vi "CC Observation List to Table.vi"(8 "error in (no error)":errorcluster, 11 "Observation List":T2[](array[typedef])) -> (0 "error out":errorcluster, 1 "Screen Ready Table":string[][](array[string]), 2 "Status":T1[](array[typedef]), 3 "File Ready Table":string[][](array[string]))   [LabVIEW 2024]
uses:
  typedefs/CC cluster Observation.ctl
  Observation Queue/CC enum Observation Status.ctl
  Telescope/CC cluster Telescope Offsets.ctl
  typedefs/CC cluster Observation Dither Options.ctl
  typedefs/CC enum Dither Selection.ctl
  typedefs/CC cluster RA and DEC.ctl
panel:
  out "Header":string[](array[string])
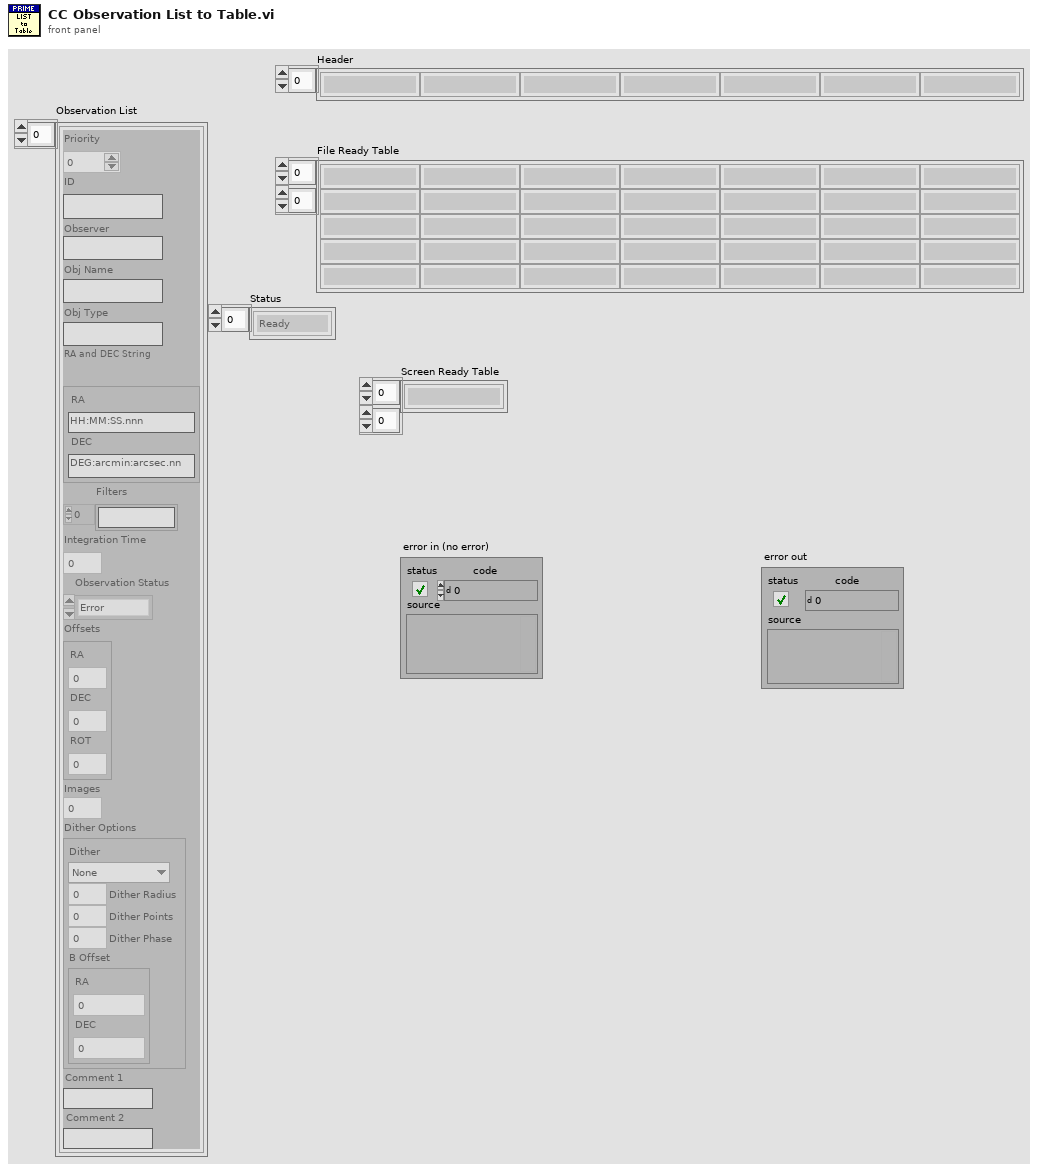
[diagram p1: front panel]
types:
  T1 = typedef "CC enum Observation Status.ctl" = enum16{"Ready", "Running", "Done", "Error"}
  T2 = typedef "CC cluster Observation.ctl" = cluster{"Priority":i32, "ID":string, "Observer":string, "Obj Name":string, "Obj Type":string, "RA and DEC String":cluster{"RA":string, "DEC":string}, "Filters":string[], "Integration Time":dbl, "Observation Status":T1, "Offsets":T3, "Images":i32, "Dither Options":T4, "Comment 1":string, "Comment 2":string}
  T3 = typedef "CC cluster Telescope Offsets.ctl" = cluster{"RA":dbl, "DEC":dbl, "ROT":dbl}
  T4 = typedef "CC cluster Observation Dither Options.ctl" = cluster{"Dither":T5, "Dither Radius":dbl, "Dither Points":i32, "Dither Phase":dbl, "B Offset":T6}
  T5 = typedef "CC enum Dither Selection.ctl" = enum16{"None", "Circle", "Random", "ABBA"}
  T6 = typedef "CC cluster RA and DEC.ctl" = cluster{"RA":dbl, "DEC":dbl}
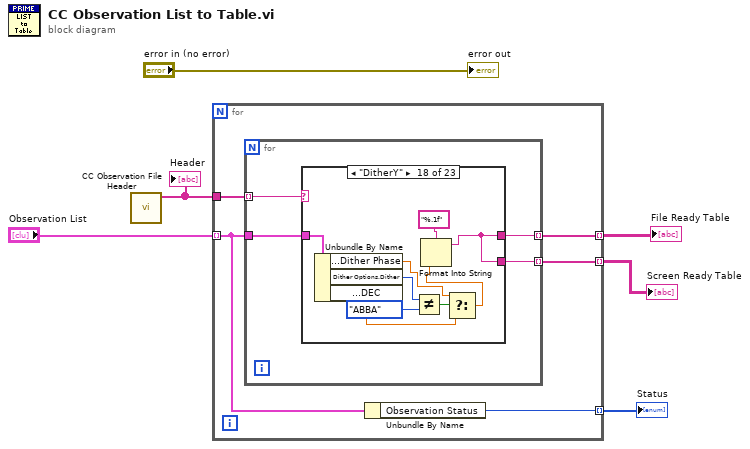
[diagram p0: block diagram]
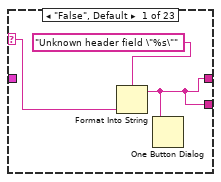
[diagram p2: hidden frame]
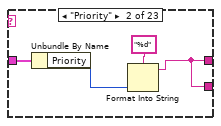
[diagram p3: hidden frame]
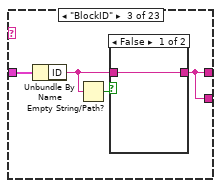
[diagram p4: hidden frame]
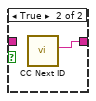
[diagram p5: hidden frame]
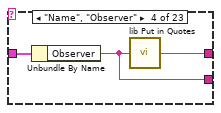
[diagram p6: hidden frame]
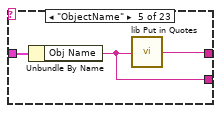
[diagram p7: hidden frame]
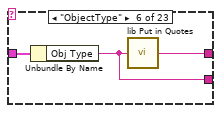
[diagram p8: hidden frame]
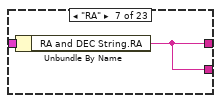
[diagram p9: hidden frame]
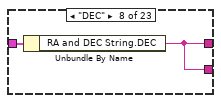
[diagram p10: hidden frame]
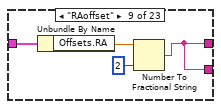
[diagram p11: hidden frame]
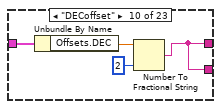
[diagram p12: hidden frame]
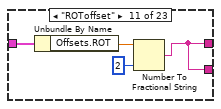
[diagram p13: hidden frame]
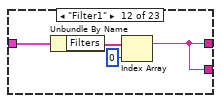
[diagram p14: hidden frame]
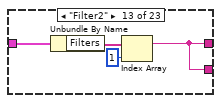
[diagram p15: hidden frame]
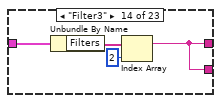
[diagram p16: hidden frame]
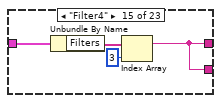
[diagram p17: hidden frame]
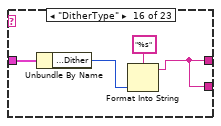
[diagram p18: hidden frame]
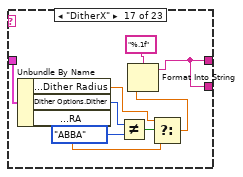
[diagram p19: hidden frame]
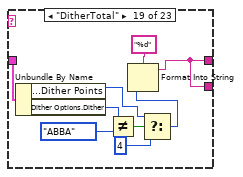
[diagram p20: hidden frame]
diagram:
  n1 = call "CC Observation File Header.vi"() -> ("Header"=w5:string[])  [unwired: 10 in, 1 out]
  "Header" <- w5
  n2 = for {
    tunnel: w5 -> [w11]
    tunnel: "Observation List" -> [w9] mode=indexing
    tunnel: [w10] -> w3 mode=indexing
    tunnel: [w8] -> w4 mode=indexing
    tunnel: [w7] -> w1 mode=indexing
    n3 = for {
      tunnel: w11 -> [w15] mode=indexing
      tunnel: w9 -> [w14]
      tunnel: [w13] -> w10 mode=indexing
      tunnel: [w12] -> w7 mode=indexing
      n4 = case shown="\"DitherY\"" w15 {
        selector: w15 -> [w17 _ _ _ _ _ _ _ _ _ _ _ _ _ _ _ _ _ _ _ _ _ _]
        tunnel: w14 -> [_ w22 w26 w31 w34 w37 w39 w41 w45 w49 w53 w57 w61 w65 w69 w73 w82 w85 w100 w104 w108 w111 w114]
        tunnel: [w16 w19 w23 w30 w33 w36 w38 w40 w42 w46 w50 w55 w59 w63 w67 w70 w80 w90 w98 w101 w105 w109 w112] -> w13
        tunnel: [w16 w19 w23 w29 w32 w35 w38 w40 w42 w46 w50 w55 w59 w63 w67 w70 w80 w90 w98 w101 w105 w109 w112] -> w12
        frame "False", Default {
          n5 = Format Into String(format string="Unknown header field \"%s\"" ("Filter Wheel 2"), w17) -> (resulting string=w16:string)  [unwired: 2 in, 1 out]
          n6 = One Button Dialog(message=w16) -> ()  [unwired: 1 in, 1 out]
        }
        frame "Priority" {
          n7 = Unbundle By Name(w22) -> ("Priority"=w20:i32)
          n8 = Format Into String(format string="%d", w20) -> (resulting string=w19:string)  [unwired: 2 in, 1 out]
        }
        frame "BlockID" {
          n9 = Unbundle By Name(w26) -> ("ID"=w24:string)
          n10 = Empty String/Path?(string/path=w24) -> (empty?=w25:bool)
          n11 = case shown="False" w25 {
            tunnel: [w27 w28] -> w23
            tunnel: w24 -> [w27 _]
            frame False {
            }
            frame True {
              n12 = call "CC Next ID.vi"() -> ("BlockID string"=w28:string)  [unwired: 9 in, 2 out]
            }
          }
        }
        frame "Name", "Observer" {
          n13 = Unbundle By Name(w31) -> ("Observer"=w29:string)
          n14 = call "lib Put in Quotes.vi"("String"=w29) -> ("Quoted String"=w30:string)  [unwired: 4 in]
        }
        frame "ObjectName" {
          n15 = Unbundle By Name(w34) -> ("Obj Name"=w32:string)
          n16 = call "lib Put in Quotes.vi"("String"=w32) -> ("Quoted String"=w33:string)  [unwired: 4 in]
        }
        frame "ObjectType" {
          n17 = Unbundle By Name(w37) -> ("Obj Type"=w35:string)
          n18 = call "lib Put in Quotes.vi"("String"=w35) -> ("Quoted String"=w36:string)  [unwired: 4 in]
        }
        frame "RA" {
          n19 = Unbundle By Name(w39) -> ("RA and DEC String.RA"=w38:string)
        }
        frame "DEC" {
          n20 = Unbundle By Name(w41) -> ("RA and DEC String.DEC"=w40:string)
        }
        frame "RAoffset" {
          n21 = Unbundle By Name(w45) -> ("Offsets.RA"=w44:dbl)
          n22 = Number To Fractional String(number=w44, precision (6)=i16 2) -> (F-format string=w42:string)  [unwired: 2 in]
        }
        frame "DECoffset" {
          n23 = Unbundle By Name(w49) -> ("Offsets.DEC"=w48:dbl)
          n24 = Number To Fractional String(number=w48, precision (6)=i16 2) -> (F-format string=w46:string)  [unwired: 2 in]
        }
        frame "ROToffset" {
          n25 = Unbundle By Name(w53) -> ("Offsets.ROT"=w52:dbl)
          n26 = Number To Fractional String(number=w52, precision (6)=i16 2) -> (F-format string=w50:string)  [unwired: 2 in]
        }
        frame "Filter1" {
          n27 = Unbundle By Name(w57) -> ("Filters"=w56:string[])
          n28 = Index Array(array=w56, index=0) -> (element=w55:string)
        }
        frame "Filter2" {
          n29 = Unbundle By Name(w61) -> ("Filters"=w60:string[])
          n30 = Index Array(array=w60, index=1) -> (element=w59:string)
        }
        frame "Filter3" {
          n31 = Unbundle By Name(w65) -> ("Filters"=w64:string[])
          n32 = Index Array(array=w64, index=2) -> (element=w63:string)
        }
        frame "Filter4" {
          n33 = Unbundle By Name(w69) -> ("Filters"=w68:string[])
          n34 = Index Array(array=w68, index=3) -> (element=w67:string)
        }
        frame "DitherType" {
          n35 = Unbundle By Name(w73) -> ("Dither Options.Dither"=w71:T5)
          n36 = Format Into String(format string="%s", w71) -> (resulting string=w70:string)  [unwired: 2 in, 1 out]
        }
        frame "DitherX" {
          n37 = Unbundle By Name(w82) -> ("Dither Options.Dither Radius"=w76:dbl, "Dither Options.Dither"=w79:T5, "Dither Options.B Offset.RA"=w74:dbl)
          n38 = Not Equal?(x=w79, y=CC_enum_Dither_Selection."ABBA") -> (x != y?=w77:bool)
          n39 = Select(t=w76, s=w77, f=w74) -> (s? t:f=w75:dbl)
          n40 = Format Into String(format string="%.1f", w75) -> (resulting string=w80:string)  [unwired: 2 in, 1 out]
        }
        frame "DitherY" {
          n41 = Unbundle By Name(w85) -> ("Dither Options.Dither Phase"=w84:dbl, "Dither Options.Dither"=w89:T5, "Dither Options.B Offset.DEC"=w86:dbl)
          n42 = Not Equal?(x=w89, y=CC_enum_Dither_Selection."ABBA") -> (x != y?=w87:bool)
          n43 = Select(t=w84, s=w87, f=w86) -> (s? t:f=w83:dbl)
          n44 = Format Into String(format string="%.1f", w83) -> (resulting string=w90:string)  [unwired: 2 in, 1 out]
        }
        frame "DitherTotal" {
          n45 = Unbundle By Name(w100) -> ("Dither Options.Dither Points"=w95:i32, "Dither Options.Dither"=w97:T5)
          n46 = Not Equal?(x=w97, y=CC_enum_Dither_Selection."ABBA") -> (x != y?=w92:bool)
          n47 = Select(t=w95, s=w92, f=4) -> (s? t:f=w94:i32)
          n48 = Format Into String(format string="%d", w94) -> (resulting string=w98:string)  [unwired: 2 in, 1 out]
        }
        frame "Images" {
          n49 = Unbundle By Name(w104) -> ("Images"=w102:i32)
          n50 = Format Into String(format string="%d", w102) -> (resulting string=w101:string)  [unwired: 2 in, 1 out]
        }
        frame "IntegrationTime" {
          n51 = Unbundle By Name(w108) -> ("Integration Time"=w106:dbl)
          n52 = Format Into String(format string="%.2f", w106) -> (resulting string=w105:string)  [unwired: 2 in, 1 out]
        }
        frame "Comment1" {
          n53 = Unbundle By Name(w111) -> ("Comment 1"=w110:string)
          n54 = call "lib Put in Quotes.vi"("String"=w110) -> ("Quoted String"=w109:string)  [unwired: 4 in]
        }
        frame "Comment2" {
          n55 = Unbundle By Name(w114) -> ("Comment 2"=w113:string)
          n56 = call "lib Put in Quotes.vi"("String"=w113) -> ("Quoted String"=w112:string)  [unwired: 4 in]
        }
      }
    }
    n57 = Unbundle By Name(w9) -> ("Observation Status"=w8:T1)
  }
  "File Ready Table" <- w3
  "Status" <- w4
  "Screen Ready Table" <- w1
  "error out" <- "error in (no error)"
